vi "ma_Spectrum Averaging (complex).vi"(3 "complex spectrum":cdb[](array[numeric]) format="%0.2p", 4 "df":dbl format="%0.2p", 7 "retrieve last spectrum (F)":bool, 8 "averaging parameters":T1={"averaging mode"=enum."No averaging", "weighting mode"=enum."Exponential", "number of averages"=10} {"number of averages" min=1}, 9 "restart averaging (F)":bool) -> (0 "averaged complex spectrum":cdb[](array[numeric]) format="%0.2p", 1 "df":dbl format="%0.2p", 5 "averaging done":bool, 6 "averages completed":dbl format="%0.2f")   [LabVIEW 2020, in "NI_MAPro.lvlib"]
uses:
  NI_MAPro.lvlib
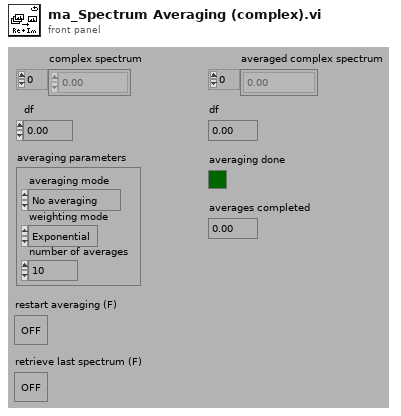
[diagram p1: front panel]
types:
  T1 = cluster{"averaging mode":enum16{"No averaging", "Vector averaging", "RMS averaging", "Peak hold"}, "weighting mode":enum16{"Linear", "Exponential"}, "number of averages":u32}
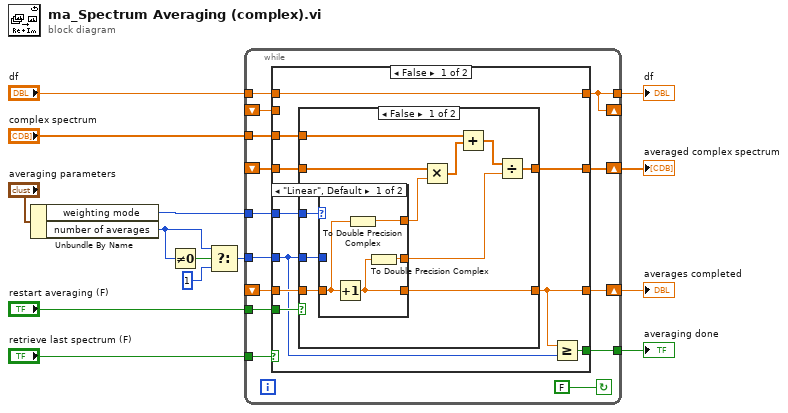
[diagram p0: block diagram]
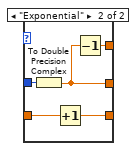
[diagram p2: hidden frame]
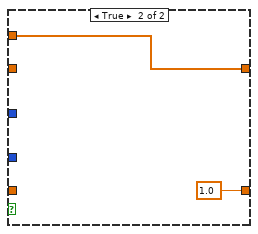
[diagram p3: hidden frame]
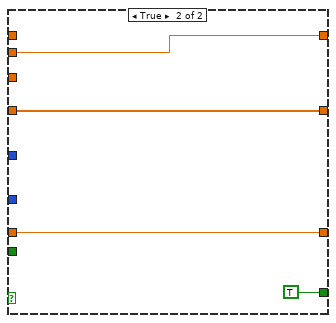
[diagram p4: hidden frame]
diagram:
  n1 = Unbundle By Name("averaging parameters") -> ("weighting mode"=w10:enum16{"Linear", "Exponential"}, "number of averages"=w3:u32)
  n2 = Not Equal To 0?(x=w3) -> (x != 0?=w4:bool)
  n3 = Select(t=w3, s=w4, f=u32 1) -> (s? t:f=w1:u32)
  n4 = while {
    shift-left: _ -> [w16]
    shift-right: [w15] -> _
    tunnel: [w15] -> w5
    tunnel: "df" -> [w17]
    tunnel: "retrieve last spectrum (F)" -> [w19]
    tunnel: [w20] -> w9
    tunnel: w1 -> [w22]
    tunnel: w10 -> [w25]
    tunnel: "complex spectrum" -> [w24]
    shift-left: _ -> [w27]
    shift-right: [w21] -> w12
    shift-left: _ -> [w26]
    shift-right: [w28] -> w8
    tunnel: "restart averaging (F)" -> [w23]
    stop <- FALSE continue-if-true
    n5 = case shown="False" w19 {
      tunnel: [w38 w64] -> w28
      tunnel: w27 -> [w37 w63]
      tunnel: w26 -> [w36 w64]
      tunnel: w25 -> [w35 _]
      tunnel: w24 -> [w34 _]
      tunnel: w23 -> [w33 _]
      tunnel: w22 -> [w32 _]
      tunnel: [w31 w63] -> w21
      tunnel: [w30 TRUE] -> w20
      tunnel: w17 -> [w29 _]
      tunnel: [w29 w61] -> w15
      tunnel: w16 -> [_ w61]
      frame False {
        n6 = case shown="False" w33 {
          tunnel: [w46 w59] -> w38
          tunnel: [w41 1.0] -> w31
          tunnel: w37 -> [w44 _]
          tunnel: w36 -> [w49 _]
          tunnel: w34 -> [w45 w59]
          tunnel: w35 -> [w42 _]
          tunnel: w32 -> [w39 _]
          frame False {
            n7 = case shown="\"Linear\", Default" w42 {
              tunnel: w44 -> [w52 w57]
              tunnel: [w50 w58] -> w41
              tunnel: [w53 w54] -> w43
              tunnel: [w51 w55] -> w40
              tunnel: w39 -> [_ w56]
              frame "Linear", Default {
                n8 = Increment(x=w52) -> (x+1=w50:dbl)
                n9 = To Double Precision Complex(1:w52) -> (0:w53:cdb)
                n10 = To Double Precision Complex(1:w50) -> (0:w51:cdb)
              }
              frame "Exponential" {
                n11 = To Double Precision Complex(1:w56) -> (0:w55:cdb)
                n12 = Increment(x=w57) -> (x+1=w58:dbl)
                n13 = Decrement(x=w55) -> (x-1=w54:cdb)
              }
            }
            n14 = Multiply(x=w49, y=w43) -> (x*y=w48:cdb[])
            n15 = Add(x=w45, y=w48) -> (x+y=w47:cdb[])
            n16 = Divide(x=w47, y=w40) -> (x/y=w46:cdb[])
          }
          frame True {
          }
        }
        n17 = Greater Or Equal?(x=w31, y=w32) -> (x >= y?=w30:bool)
      }
      frame True {
      }
    }
  }
  "averaged complex spectrum" <- w8
  "averages completed" <- w12
  "averaging done" <- w9
  "df" <- w5
